vi "laser_controller.vi"() -> ()   [LabVIEW 2014]
uses:
  <vilib>/Instr/_visa.llb/VISA Configure Serial Port (Instr).vi
  <vilib>/FieldPoint/Polymorphic Read.llb/FP Read (Float Array).vi
  <vilib>/FieldPoint/Polymorphic Write.llb/FP Write (Float).vi
panel:
  in  "Change Power?":bool
  out "TEC Setpoint":dbl format="%#_13g"
  out "Power":dbl(graph)
  in  "DISABLE":bool
  in  "ENABLE":bool
  in  "LEVEL CONTROL, 0-100 (%)":dbl(knob) scale=0.0..100.0
  out "Temp":dbl(graph)
  in  "Which Temp?":enum16{"ETH", "PUMP", "PCB", "AMP", "CASE"}(ring)
  out "Temp Stable":bool=TRUE
  out "Software Enabled":bool=TRUE
  out "Hardware Enabled":bool=TRUE
  in  "Ethernal COM Port":refnum<visa-resource-name>="COM1"
  in  "LEVEL CONTROL, 0-10 (W)":dbl(knob) scale=0.0..10.0
  in  "AMPLIFIER ENABLE":bool
  out "Pre-amp Mon (Amps)":dbl format="%#_3g"
  out "Temp Mon (deg C)":dbl(slide) scale=0.0..50.0
  out "Mid Power Mon (Volts, no-cal)":dbl format="%#_3g"
  out "Out Power Mon (Volts, no-cal)":dbl format="%#_3g"
  out "+5 Vdc Out":dbl format="%#_3g"
  out "Power-Amp Pump Current (Amps)":dbl format="%#_3g"
  out "Seed Mon (Volts, no-cal)":dbl format="%#_3g"
  out "Back Refl. Mon (Volts, no-cal)":dbl format="%#_3g"
  out "Power Supply Fault":bool=TRUE
  out "Temp. Fault":bool=TRUE
  out "Back Refl. Fault":bool=TRUE
  out "Seed Power Fault":bool=TRUE
  out "Master Fault":bool=TRUE
  in  "Controller Stop":bool
  in  "Control Rate (ms)":u32=290
  # "ORBITS SEED LASER"
  # "NUFERN FIBER AMPLIFIER"
  # "STATUS"
  # "FAULT STATUS"
  # "MONITORS"
  # "OFF STATUS"
  # "ON STATUS"
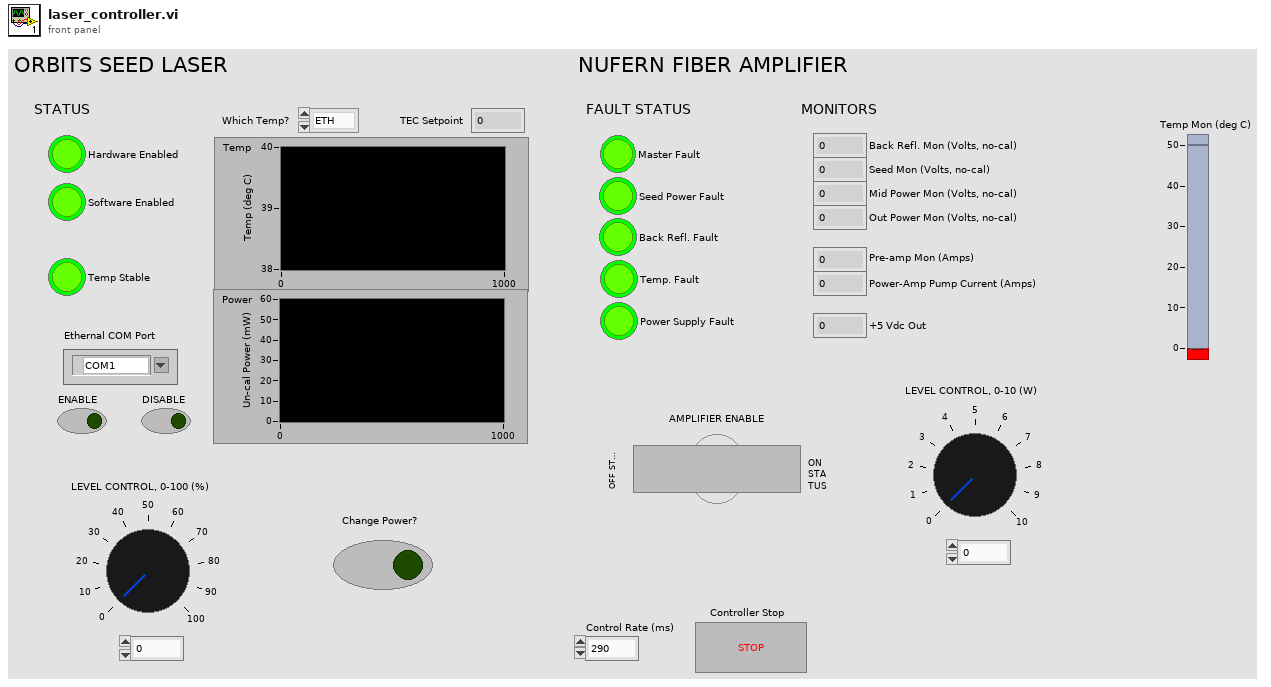
[diagram p1: front panel]
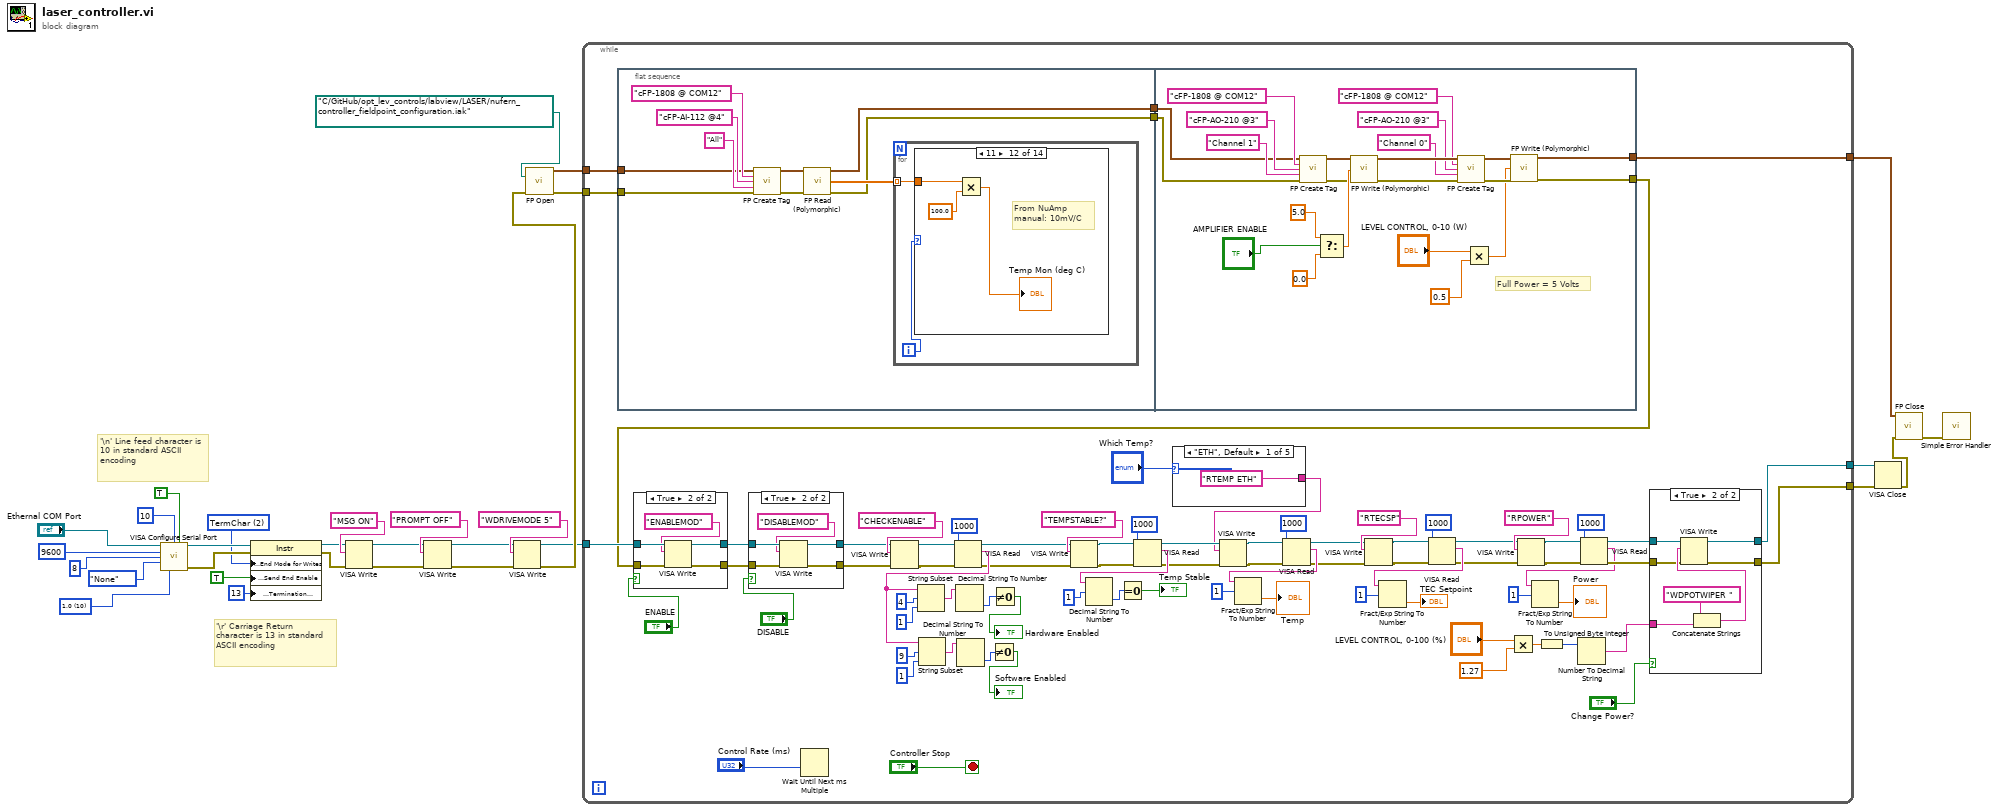
[diagram p0: block diagram]
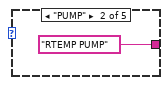
[diagram p5: hidden frame]
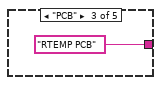
[diagram p6: hidden frame]
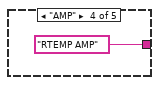
[diagram p7: hidden frame]
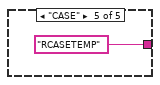
[diagram p8: hidden frame]
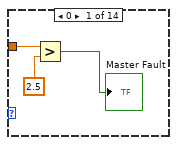
[diagram p9: hidden frame]
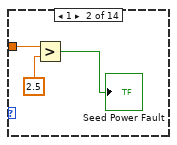
[diagram p10: hidden frame]
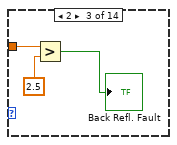
[diagram p11: hidden frame]
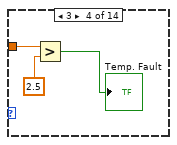
[diagram p12: hidden frame]
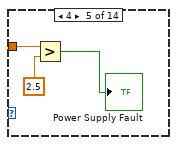
[diagram p13: hidden frame]
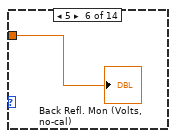
[diagram p14: hidden frame]
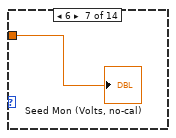
[diagram p15: hidden frame]
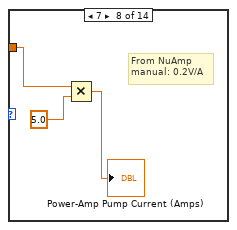
[diagram p16: hidden frame]
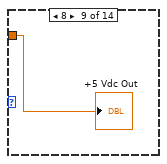
[diagram p17: hidden frame]
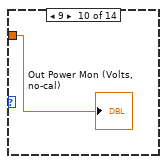
[diagram p18: hidden frame]
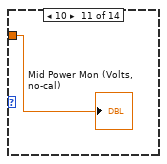
[diagram p19: hidden frame]
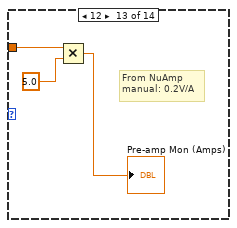
[diagram p20: hidden frame]
diagram:
  w6 = u16 10 items=["1.0"=10, "1.5"=15, "2.0"=20] ("stop bits (10: 1 bit)")
  w23 = u16 2 items=["None", "LastBit", "TermChar", "Break"] ("Serial Settings:Serial End Mode for Writes")
  # "'\\r' Carriage Return character is 13 in standard ASCII encoding"
  # "'\\n' Line feed character is 10 in standard ASCII encoding"
  n1 = call-poly "VISA Configure Serial Port"("VISA resource name"="Ethernal COM Port", "termination char\n(0xA = '\\n' = LF)"=u8 10, "Enable Termination\nChar (T)"=TRUE, "baud rate (9600)"=u32 9600, "data bits (8)"=u16 8, "parity (0:none)"=enum16{"None", "Odd", "Even", "Mark", "Space"}."None", "stop bits (10: 1 bit)"=w6) -> ("VISA resource name out"=w25:refnum<visa-resource-name>, "error out"=w26:errorcluster)  [unwired: 3 in, 4 out]
  n2 = property class="Instr"(reference=w25, error in=w26, "Serial Settings:End Mode for Writes"=w23, "Message Based Settings:Send End Enable"=TRUE, "Message Based Settings:Termination Character"=13) -> (reference out=w13:refnum<visa-resource-name>, error out=w14:errorcluster)
  n3 = VISA Write(VISA resource name=w13, write buffer="MSG ON" ("Enable 2"), error in (no error)=w14) -> (VISA resource name out=w11:refnum<visa-resource-name>, error out=w10:errorcluster)  [unwired: 1 out]
  n4 = VISA Write(VISA resource name=w11, write buffer="PROMPT OFF" ("Enable 2"), error in (no error)=w10) -> (VISA resource name out=w4:refnum<visa-resource-name>, error out=w3:errorcluster)  [unwired: 1 out]
  n5 = VISA Write(VISA resource name=w4, write buffer="WDRIVEMODE 5" ("Enable 2"), error in (no error)=w3) -> (VISA resource name out=w1:refnum<visa-resource-name>, error out=w2:errorcluster)  [unwired: 1 out]
  n6 = call <vilib>:"FP Open.vi"("iak file path"=path "C:/GitHub/opt_lev_controls/labview/LASER/nufern_controller_fieldpoint_configuration.iak", "error in (no error)"=w2) -> ("FP refnum out"=w31:cluster{"server refnum":u32, "tag refnum":u32}, "error out"=w30:errorcluster)  [unwired: 12 in]
  n7 = while {
    tunnel: w31 -> [w107]
    tunnel: w30 -> [w106]
    tunnel: [w103] -> w28
    tunnel: w1 -> [w61]
    tunnel: [w63] -> w8
    tunnel: [w62] -> w7
    stop <- "Controller Stop" stop-if-true
    n8 = flat-sequence {
      tunnel: w107 -> [w141]
      tunnel: w106 -> [w140]
      tunnel: [w139] -> w105
      tunnel: [w138] -> w104
      tunnel: w105 -> [w198]
      tunnel: w104 -> [w197]
      tunnel: [w183] -> w103
      tunnel: [w182] -> w60
      frame #0 {
        n9 = call <vilib>:"FP Create Tag.vi"("FP refnum in"=w141, "comm resource name"="cFP-1808 @ COM12" ("Comm Resource Name"), "device name"="cFP-AI-112 @4" ("Device Name"), "item name"="All" ("Item Name"), "error in (no error)"=w140) -> ("FP refnum out"=w143:cluster{"server refnum":u32, "tag refnum":u32}, "error out"=w142:errorcluster)  [unwired: 9 in]
        n10 = call-poly <vilib>:"FP Read (Polymorphic).vi"("FP refnum in"=w143, "error in (no error)"=w142) -> ("FP refnum out"=w139:cluster{"server refnum":u32, "tag refnum":u32}, "values"=w147:dbl[], "error out"=w138:errorcluster)  [unwired: 10 in, 1 out]
        n11 = for {
          tunnel: w147 -> [w149] mode=indexing
          i -> [w148]
          n12 = case shown="11" w148 {
            tunnel: w149 -> [w152 w155 w158 w161 w164 w165 w166 w169 w170 w171 w172 w174 w177 _]
            frame 0 {
              n13 = Greater?(x=w152, y=2.5) -> (0:→"Master Fault":bool)
            }
            frame 1 {
              n14 = Greater?(x=w155, y=2.5) -> (0:→"Seed Power Fault":bool)
            }
            frame 2 {
              n15 = Greater?(x=w158, y=2.5) -> (0:→"Back Refl. Fault":bool)
            }
            frame 3 {
              n16 = Greater?(x=w161, y=2.5) -> (0:→"Temp. Fault":bool)
            }
            frame 4 {
              n17 = Greater?(x=w164, y=2.5) -> (0:→"Power Supply Fault":bool)
            }
            frame 5 {
              "Back Refl. Mon (Volts, no-cal)" <- w165
            }
            frame 6 {
              "Seed Mon (Volts, no-cal)" <- w166
            }
            frame 7 {
              # "From NuAmp \nmanual: 0.2V/A"
              n18 = Multiply(x=w169, y=5.0) -> (x*y=→"Power-Amp Pump Current (Amps)":dbl)
            }
            frame 8 {
              "+5 Vdc Out" <- w170
            }
            frame 9 {
              "Out Power Mon (Volts, no-cal)" <- w171
            }
            frame 10 {
              "Mid Power Mon (Volts, no-cal)" <- w172
            }
            frame 11 {
              # "From NuAmp \nmanual: 10mV/C"
              n19 = Multiply(x=w174, y=100.0) -> (x*y=→"Temp Mon (deg C)":dbl)
            }
            frame 12 {
              # "From NuAmp \nmanual: 0.2V/A"
              n20 = Multiply(x=w177, y=5.0) -> (x*y=→"Pre-amp Mon (Amps)":dbl)
            }
            frame 13, Default {
            }
          }
        }
      }
      frame #1 {
        # "Full Power = 5 Volts"
        n21 = call <vilib>:"FP Create Tag.vi"("FP refnum in"=w198, "comm resource name"="cFP-1808 @ COM12" ("Comm Resource Name"), "device name"="cFP-AO-210 @3" ("Device Name"), "item name"="Channel 1" ("Item Name"), "error in (no error)"=w197) -> ("FP refnum out"=w192:cluster{"server refnum":u32, "tag refnum":u32}, "error out"=w191:errorcluster)  [unwired: 9 in]
        n22 = Select(t=5.0, s="AMPLIFIER ENABLE", f=0.0) -> (s? t:f=w193:dbl)
        n23 = call-poly <vilib>:"FP Write (Polymorphic).vi"("FP refnum in"=w192, "value"=w193, "error in (no error)"=w191) -> ("FP refnum out"=w190:cluster{"server refnum":u32, "tag refnum":u32}, "error out"=w189:errorcluster)  [unwired: 10 in, 1 out]
        n24 = call <vilib>:"FP Create Tag.vi"("FP refnum in"=w190, "comm resource name"="cFP-1808 @ COM12" ("Comm Resource Name"), "device name"="cFP-AO-210 @3" ("Device Name"), "item name"="Channel 0" ("Item Name"), "error in (no error)"=w189) -> ("FP refnum out"=w185:cluster{"server refnum":u32, "tag refnum":u32}, "error out"=w184:errorcluster)  [unwired: 9 in]
        n25 = Multiply(x="LEVEL CONTROL, 0-10 (W)", y=0.5) -> (x*y=w179:dbl)
        n26 = call-poly <vilib>:"FP Write (Polymorphic).vi"("FP refnum in"=w185, "value"=w179, "error in (no error)"=w184) -> ("FP refnum out"=w183:cluster{"server refnum":u32, "tag refnum":u32}, "error out"=w182:errorcluster)  [unwired: 10 in, 1 out]
      }
    }
    n27 = case shown="True" "ENABLE" {
      tunnel: w61 -> [w118 w123]
      tunnel: w60 -> [w117 w122]
      tunnel: [w118 w121] -> w59
      tunnel: [w117 w120] -> w58
      frame False {
      }
      frame True {
        n28 = VISA Write(VISA resource name=w123, write buffer="ENABLEMOD" ("Enable 2"), error in (no error)=w122) -> (VISA resource name out=w121:refnum<visa-resource-name>, error out=w120:errorcluster)  [unwired: 1 out]
      }
    }
    n29 = case shown="True" "DISABLE" {
      tunnel: w59 -> [w111 w116]
      tunnel: w58 -> [w110 w115]
      tunnel: [w111 w114] -> w57
      tunnel: [w110 w113] -> w56
      frame False {
      }
      frame True {
        n30 = VISA Write(VISA resource name=w116, write buffer="DISABLEMOD" ("Enable 2"), error in (no error)=w115) -> (VISA resource name out=w114:refnum<visa-resource-name>, error out=w113:errorcluster)  [unwired: 1 out]
      }
    }
    n31 = Wait Until Next ms Multiple(millisecond multiple="Control Rate (ms)") -> ()  [unwired: 1 out]
    n32 = VISA Write(VISA resource name=w57, write buffer="CHECKENABLE" ("Enable 2"), error in (no error)=w56) -> (VISA resource name out=w100:refnum<visa-resource-name>, error out=w99:errorcluster)  [unwired: 1 out]
    n33 = VISA Read(VISA resource name=w100, byte count=u32 1000 ("Read Count"), error in (no error)=w99) -> (VISA resource name out=w82:refnum<visa-resource-name>, read buffer=w94:string, error out=w81:errorcluster)  [unwired: 1 out]
    n34 = String Subset(string=w94, offset (0)=4, length (rest)=1) -> (substring=w93:string)
    n35 = String Subset(string=w94, offset (0)=9, length (rest)=1) -> (substring=w92:string)
    n36 = Decimal String To Number(string=w93) -> (number=w91:i32)  [unwired: 2 in, 1 out]
    n37 = Decimal String To Number(string=w92) -> (number=w88:i32)  [unwired: 2 in, 1 out]
    n38 = Not Equal To 0?(x=w88) -> (x != 0?=→"Software Enabled":bool)
    n39 = Not Equal To 0?(x=w91) -> (x != 0?=→"Hardware Enabled":bool)
    n40 = VISA Write(VISA resource name=w82, write buffer="TEMPSTABLE?" ("Enable 2"), error in (no error)=w81) -> (VISA resource name out=w85:refnum<visa-resource-name>, error out=w84:errorcluster)  [unwired: 1 out]
    n41 = VISA Read(VISA resource name=w85, byte count=u32 1000 ("Read Count 3"), error in (no error)=w84) -> (VISA resource name out=w74:refnum<visa-resource-name>, read buffer=w83:string, error out=w73:errorcluster)  [unwired: 1 out]
    n42 = Decimal String To Number(string=w83, offset=1) -> (number=w79:i32)  [unwired: 1 in, 1 out]
    n43 = Equal To 0?(x=w79) -> (x = 0?=→"Temp Stable":bool)
    n44 = case shown="\"ETH\", Default" "Which Temp?" {
      tunnel: ["RTEMP ETH" ("Enable 2") "RTEMP PUMP" ("Enable 2") "RTEMP PCB" ("Enable 2") "RTEMP AMP" ("Enable 2") "RCASETEMP" ("Enable 2")] -> w72
      frame "ETH", Default {
      }
      frame "PUMP" {
      }
      frame "PCB" {
      }
      frame "AMP" {
      }
      frame "CASE" {
      }
    }
    n45 = VISA Write(VISA resource name=w74, write buffer=w72, error in (no error)=w73) -> (VISA resource name out=w76:refnum<visa-resource-name>, error out=w75:errorcluster)  [unwired: 1 out]
    n46 = VISA Read(VISA resource name=w76, byte count=u32 1000 ("Read Count 3"), error in (no error)=w75) -> (VISA resource name out=w42:refnum<visa-resource-name>, read buffer=w71:string, error out=w41:errorcluster)  [unwired: 1 out]
    n47 = Fract/Exp String To Number(string=w71, offset=1) -> (number=→"Temp":dbl)  [unwired: 2 in, 1 out]
    n48 = VISA Write(VISA resource name=w42, write buffer="RTECSP" ("Enable 2"), error in (no error)=w41) -> (VISA resource name out=w47:refnum<visa-resource-name>, error out=w46:errorcluster)  [unwired: 1 out]
    n49 = VISA Read(VISA resource name=w47, byte count=u32 1000 ("Read Count 3"), error in (no error)=w46) -> (VISA resource name out=w40:refnum<visa-resource-name>, read buffer=w43:string, error out=w39:errorcluster)  [unwired: 1 out]
    n50 = Fract/Exp String To Number(string=w43, offset=1) -> (number=→"TEC Setpoint":dbl)  [unwired: 2 in, 1 out]
    n51 = Multiply(x="LEVEL CONTROL, 0-100 (%)", y=1.27) -> (x*y=w34:dbl)
    n52 = VISA Write(VISA resource name=w40, write buffer="RPOWER" ("Enable 2"), error in (no error)=w39) -> (VISA resource name out=w68:refnum<visa-resource-name>, error out=w67:errorcluster)  [unwired: 1 out]
    n53 = To Unsigned Byte Integer(number=w34) -> (unsigned 8bit integer=w33:u8)
    n54 = Number To Decimal String(number=w33) -> (decimal integer string=w32:string)  [unwired: 1 in]
    n55 = VISA Read(VISA resource name=w68, byte count=u32 1000 ("Read Count 3"), error in (no error)=w67) -> (VISA resource name out=w65:refnum<visa-resource-name>, read buffer=w50:string, error out=w64:errorcluster)  [unwired: 1 out]
    n56 = Fract/Exp String To Number(string=w50, offset=1) -> (number=→"Power":dbl)  [unwired: 2 in, 1 out]
    n57 = case shown="True" "Change Power?" {
      tunnel: w32 -> [_ w131]
      tunnel: w65 -> [w125 w129]
      tunnel: w64 -> [w124 w128]
      tunnel: [w125 w127] -> w63
      tunnel: [w124 w126] -> w62
      frame False {
      }
      frame True {
        n58 = Concatenate Strings("WDPOTWIPER " ("Enable 2"), w131) -> (w130:string)
        n59 = VISA Write(VISA resource name=w129, write buffer=w130, error in (no error)=w128) -> (VISA resource name out=w127:refnum<visa-resource-name>, error out=w126:errorcluster)  [unwired: 1 out]
      }
    }
  }
  n60 = VISA Close(VISA resource name=w8, error in (no error)=w7) -> (error out=w16:errorcluster)
  n61 = call <vilib>:"FP Close.vi"("FP refnum in"=w28, "error in (no error)"=w16) -> ("error out"=w29:errorcluster)  [unwired: 13 in]
  n62 = call <vilib>:"Simple Error Handler.vi"("error in (no error)"=w29) -> ()  [unwired: 4 in, 5 out]
